vi "CalculosParametros.vi"(0 "2D Array":dbl[][](array[numeric]), 1 "Frecuencia \nMuestreo":dbl=5000.0 format="%#_13g") -> (2 "output cluster":T2, 3 "Voltaje":T1, 4 "Corriente":T1)   [LabVIEW 2014]
uses:
  <vilib>/Analysis/5stat.llb/RMS (DBL).vi
  <vilib>/Analysis/baseanly.llb/Mean (DBL).vi
  <vilib>/measure/mascope.llb/Amplitude and Levels 1 chan.vi
  <vilib>/measure/matone.llb/Harmonic Distortion Analyzer 1 Chan.vi
  <vilib>/Analysis/NI_AALPro.lvlib
  <vilib>/Analysis/NI_AALBase.lvlib
  <vilib>/measure/NI_MAPro.lvlib
panel:
  in  "Ajuste de ganancia I":dbl=1.0 format="%#_13g"
  in  "Ajuste de ganancia V":dbl=102.28846559570813 format="%#_13g"
  out "Ip-":dbl format="%.4g"
  out "Ip+":dbl format="%.4g"
  out "Corriete pp":dbl format="%.4p"
  out "Vp-":dbl format="%.4g"
  out "Vp+":dbl format="%.4g"
  out "Voltaje pp":dbl format="%.6p"
  out "Desfasaje prom":dbl
  out "THD I":dbl format="%.2p"
  out "THD V":dbl format="%.2p"
  out "Potencia Reactiva":dbl
  out "FDP":dbl
  out "Potencia Aparente":dbl format="%0.2f"
  out "Frecuencia":dbl format="%.2p"
  out "Potencia \nActiva":dbl format="%0.2f"
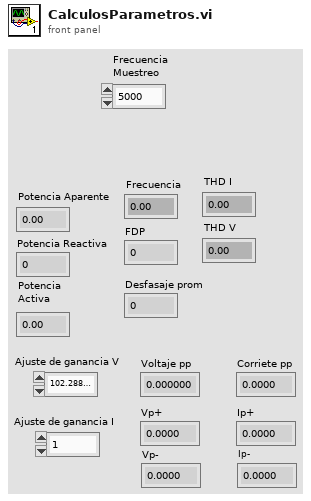
[diagram p1: front panel]
types:
  T1 = cluster{"components level":dbl[], "exported spectrum (dB)":cluster{"f0":dbl, "df":dbl, "dB Spectrum (Hann)":dbl[]}, "Waveform":waveform(dbl), "Power Spectrum (V^2 rms)":dbl[]}
  T2 = cluster{"Frecuencia":dbl, "THD V":dbl, "THD I":dbl, "FDP":dbl, "Potencia Activa":dbl, "Potencia Reactiva":dbl, "Potencia Aparente":dbl, "Desfasaje (FDP)":dbl, "Desfasaje (TM)":dbl, "Flujo":dbl, "Vrms":dbl, "Irms":dbl, "Energia":dbl}
  T3 = enum16{"none", "input signal", "fundamental signal", "residual signal", "harmonics only", "noise and spurs"}
  T4 = cluster{"exported time signal":waveform(dbl), "exported spectrum (dB)":cluster{"f0":dbl, "df":dbl, "dB Spectrum (Hann)":dbl[]}}
  T5 = cluster{"f0":dbl, "df":dbl, "dB Spectrum (Hann)":dbl[]}
  T6 = cluster{"components level":dbl[], "exported spectrum (dB)":cluster{"f0":dbl, "df":dbl, "dB Spectrum (Hann)":dbl[]}, waveform(dbl), "Power Spectrum (V^2 rms)":dbl[]}
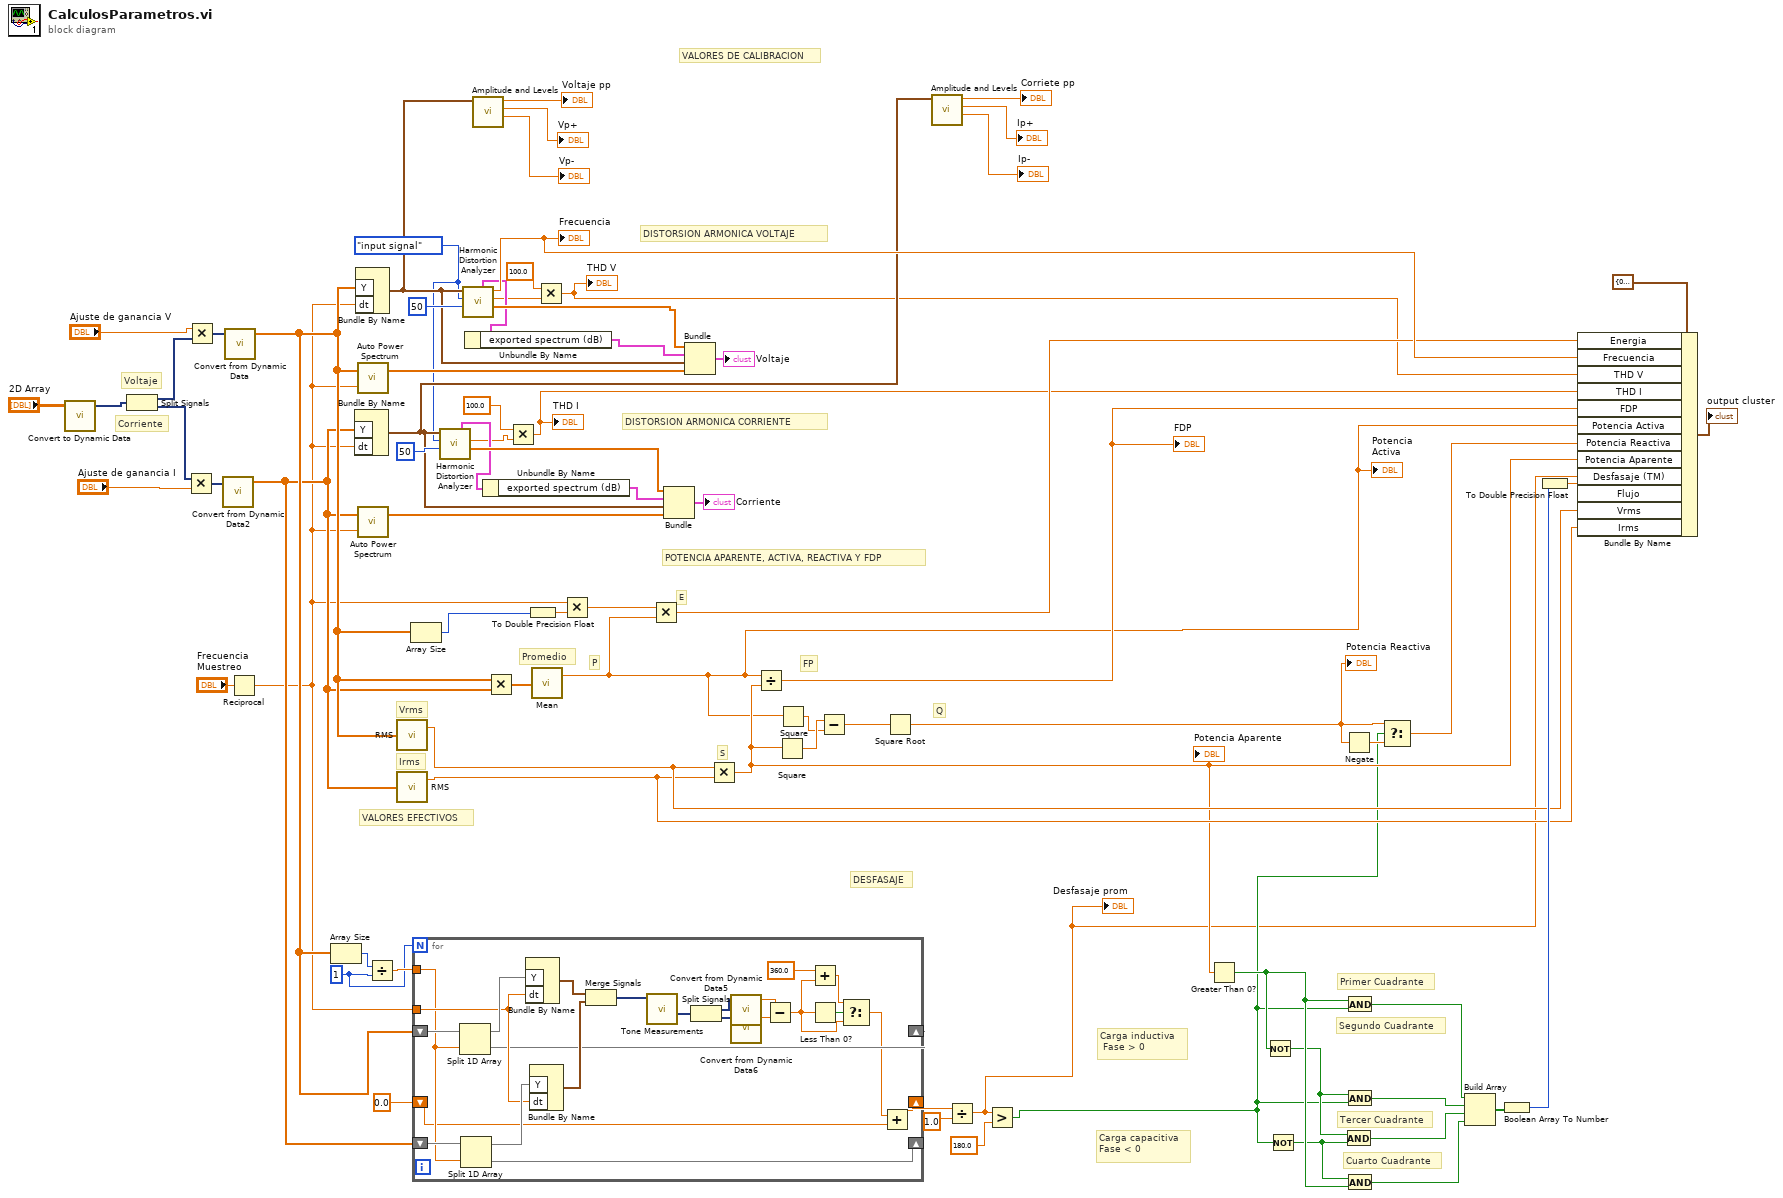
[diagram p0: block diagram]
diagram:
  w11 = T3."input signal" ("export mode")
  w47 = 1
  # "FP"
  # "VALORES EFECTIVOS"
  # "VALORES DE CALIBRACION"
  # "S"
  # "E"
  # "Q"
  # "P"
  # "Carga capacitiva \nFase < 0"
  # "Carga inductiva \n Fase > 0"
  # "Cuarto Cuadrante"
  # "Tercer Cuadrante"
  # "Segundo Cuadrante"
  # "Primer Cuadrante"
  # "DISTORSION ARMONICA VOLTAJE"
  # "DISTORSION ARMONICA CORRIENTE"
  # "Promedio"
  # "POTENCIA APARENTE, ACTIVA, REACTIVA Y FDP"
  # "Vrms"
  # "Irms"
  # "DESFASAJE"
  # "Corriente"
  # "Voltaje"
  n1 = call "Convert to Dynamic Data"("2D Array"="2D Array") -> ("Dynamic Data Type"=w55:dynamicdata)  [unwired: 3 in]
  n2 = Split Signals(w55) -> (w54:dynamicdata, w46:dynamicdata)  [unwired: 2 in]
  n3 = Multiply(x=w46, y="Ajuste de ganancia I") -> (x*y=w45:dynamicdata)
  n4 = Multiply(x="Ajuste de ganancia V", y=w54) -> (x*y=w53:dynamicdata)
  n5 = call "Convert from Dynamic Data2"("Dynamic Data Type"=w45) -> ("Array"=w21:dbl[])  [unwired: 3 in]
  n6 = call "Convert from Dynamic Data"("Dynamic Data Type"=w53) -> ("Array"=w22:dbl[])  [unwired: 3 in]
  n7 = Reciprocal(x="Frecuencia \nMuestreo") -> (1/x=w20:dbl)
  n8 = Array Size(array=w22) -> (size(s)=w48:i32)
  n9 = Bundle By Name("Y"=w21, "dt"=w20) -> (w23:waveform(dbl))  [unwired: 1 in]
  n10 = Bundle By Name("Y"=w22, "dt"=w20) -> (w30:waveform(dbl))  [unwired: 1 in]
  n11 = call <vilib>:"Auto Power Spectrum.vi"("dt"=w20, "Signal (V)"=w22) -> ("Power Spectrum (V^2 rms)"=w75:dbl[])  [unwired: 1 out]
  n12 = call <vilib>:"Auto Power Spectrum.vi"("dt"=w20, "Signal (V)"=w21) -> ("Power Spectrum (V^2 rms)"=w74:dbl[])  [unwired: 1 out]
  n13 = Divide(x=w48, y=w47) -> (x/y=w49:dbl)
  n14 = call-poly <vilib>:"RMS.vi"("X"=w22) -> ("rms value"=w62:dbl)  [unwired: 1 out]
  n15 = call-poly <vilib>:"RMS.vi"("X"=w21) -> ("rms value"=w61:dbl)  [unwired: 1 out]
  n16 = Array Size(array=w22) -> (size(s)=w39:i32)
  n17 = for {
    N: w47 -> [_]
    shift-right: [w87] -> _
    shift-left: w22 -> [w100]
    tunnel: w20 -> [w96]
    shift-right: [w83] -> _
    shift-left: w21 -> [w97]
    shift-right: [w89] -> w4
    shift-left: 0.0 -> [w84]
    tunnel: w49 -> [w85]
    n18 = Split 1D Array(array=w100, index=w85) -> (first subarray=w99:dbl[], second subarray=w87:dbl[])
    n19 = Split 1D Array(array=w97, index=w85) -> (first subarray=w98:dbl[], second subarray=w83:dbl[])
    n20 = Bundle By Name ("Build Waveform")("Y"=w99, "dt"=w96) -> (w86:waveform(dbl))  [unwired: 1 in]
    n21 = Bundle By Name("Y"=w98, "dt"=w96) -> (w95:waveform(dbl))  [unwired: 1 in]
    n22 = Merge Signals(w86, w95) -> (w88:dynamicdata)
    n23 = call "Tone Measurements"("Signals"=w88) -> ("Phase"=w91:dynamicdata)  [unwired: 9 in, 1 out]
    n24 = Split Signals(w91) -> (w90:dynamicdata, w94:dynamicdata)  [unwired: 2 in]
    n25 = call "Convert from Dynamic Data5"("Dynamic Data Type"=w90) -> ("Scalar"=w93:dbl)  [unwired: 3 in]
    n26 = call "Convert from Dynamic Data6"("Dynamic Data Type"=w94) -> ("Scalar"=w92:dbl)  [unwired: 3 in]
    n27 = Subtract(x=w93, y=w92) -> (x-y=w78:dbl)
    n28 = Add(x=360.0 ("y"), y=w78) -> (x+y=w80:dbl)
    n29 = Less Than 0?(x=w78) -> (x < 0?=w82:bool)
    n30 = Select(t=w80, s=w82, f=w78) -> (s? t:f=w81:dbl)
    n31 = Add(x=w81, y=w84) -> (x+y=w89:dbl)
  }
  n32 = call-poly <vilib>:"Harmonic Distortion Analyzer.vi"("highest harmonic"=50, "export mode"=w11, "signal in"=w23) -> ("components level"=w16:dbl[], "THD"=w9:dbl, "exported signals"=w12:T4)  [unwired: 3 in, 3 out]
  n33 = call-poly <vilib>:"Harmonic Distortion Analyzer.vi"("highest harmonic"=50, "export mode"=w11, "signal in"=w30) -> ("components level"=w19:dbl[], "THD"=w6:dbl, "detected fundamental frequency"=w73:dbl, "exported signals"=w14:T4)  [unwired: 3 in, 2 out]
  "Frecuencia" <- w73
  n34 = Unbundle By Name(w14) -> ("exported spectrum (dB)"=w13:T5)
  n35 = call-poly <vilib>:"Amplitude and Levels.vi"("signal in"=w30) -> ("low state level"=→"Vp-":dbl, "high state level"=→"Vp+":dbl, "amplitude"=→"Voltaje pp":dbl)  [unwired: 7 in, 1 out]
  n36 = Unbundle By Name(w12) -> ("exported spectrum (dB)"=w17:T5)
  n37 = Multiply(x=w22, y=w21) -> (x*y=w77:dbl[])
  n38 = Multiply(x=100.0, y=w9) -> (x*y=w10:dbl)
  "THD I" <- w10
  n39 = To Double Precision Float(number=w39) -> (double precision float=w40:dbl)
  n40 = call-poly <vilib>:"Mean.vi"("X"=w77) -> ("mean"=w35:dbl)  [unwired: 1 out]
  "Potencia \nActiva" <- w35
  n41 = Multiply(x=100.0, y=w6) -> (x*y=w7:dbl)
  "THD V" <- w7
  n42 = Multiply(x=w20, y=w40) -> (x*y=w41:dbl)
  n43 = Multiply(x=w41, y=w35) -> (x*y=w37:dbl)
  n44 = Bundle("components level"=w16, "exported spectrum (dB)"=w17, w23, "Power Spectrum (V^2 rms)"=w74) -> (→"Corriente":T6)  [unwired: 1 in]
  n45 = Bundle("components level"=w19, "exported spectrum (dB)"=w13, w30, "Power Spectrum (V^2 rms)"=w75) -> (→"Voltaje":T6)  [unwired: 1 in]
  n46 = Multiply(x=w62, y=w61) -> (x*y=w36:dbl)
  "Potencia Aparente" <- w36
  n47 = Divide(x=w35, y=w36) -> (x/y=w64:dbl)
  "FDP" <- w64
  n48 = Square(x=w36) -> (x^2=w34:dbl)
  n49 = Square(x=w35) -> (x^2=w33:dbl)
  n50 = Subtract(x=w34, y=w33) -> (x-y=w32:dbl)
  n51 = Square Root(x=w32) -> (sqrt(x)=w31:dbl)
  "Potencia Reactiva" <- w31
  n52 = call-poly <vilib>:"Amplitude and Levels.vi"("signal in"=w23) -> ("low state level"=→"Ip-":dbl, "high state level"=→"Ip+":dbl, "amplitude"=→"Corriete pp":dbl)  [unwired: 7 in, 1 out]
  n53 = Divide(x=w4, y=1.0) -> (x/y=w1:dbl)
  "Desfasaje prom" <- w1
  n54 = Greater?(x=w1, y=180.0) -> (0:w2:bool)
  n55 = Greater Than 0?(x=w36) -> (x > 0?=w65:bool)
  n56 = Not(x=w65) -> (.not. x?=w60:bool)
  n57 = Not(x=w2) -> (.not. x?=w59:bool)
  n58 = Negate(x=w31) -> (-x=w57:dbl)
  n59 = And(x=w60, y=w59) -> (x .and. y?=w69:bool)
  n60 = And(x=w65, y=w2) -> (x .and. y?=w71:bool)
  n61 = And(x=w60, y=w2) -> (x .and. y?=w70:bool)
  n62 = And(x=w59, y=w65) -> (x .and. y?=w68:bool)
  n63 = Select(t=w31, s=w2, f=w57) -> (s? t:f=w58:dbl)
  n64 = Build Array(w71, w70, w69, w68) -> (w67:bool[])
  n65 = Boolean Array To Number(Boolean array=w67) -> (number=w66:u32)
  n66 = To Double Precision Float(number=w66) -> (double precision float=w63:dbl)
  n67 = Bundle By Name(cluster=T2 {"Frecuencia"=0.0, "THD V"=0.0, "THD I"=0.0, "FDP"=0.0, "Potencia Activa"=0.0, "Potencia Reactiva"=0.0, "Potencia Aparente"=0.0, "Desfasaje (FDP)"=0.0, "Desfasaje (TM)"=0.0, "Flujo"=0.0, "Vrms"=0.0, "Irms"=0.0, "Energia"=0.0}, "Energia"=w37, "Frecuencia"=w73, "THD V"=w7, "THD I"=w10, "FDP"=w64, "Potencia Activa"=w35, "Potencia Reactiva"=w58, "Potencia Aparente"=w36, "Desfasaje (TM)"=w1, "Flujo"=w63, "Vrms"=w62, "Irms"=w61) -> (→"output cluster":T2)
